vi "Get Custom Device in System Definition.vi"(8 "error in (no error)":errorcluster, 11 "system definition":path) -> (0 "error out":errorcluster, 3 "Ballard ARINC 429 custom device":u64)   [LabVIEW 2020, in "Mutation.lvclass"]
uses:
  Mutation.lvclass
  NationalInstruments.VeriStand.SystemDefinitionAPI
  <vilib>/NI/VeriStand Custom Device Testing Tools/VeriStandTestUtilities/VeriStandTestUtilities.lvlib
  Scripting/Ballard/Ballard ARINC 429 Scripting.lvlib
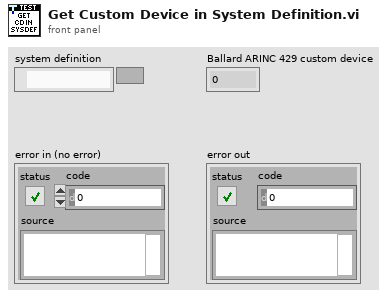
[diagram p1: front panel]
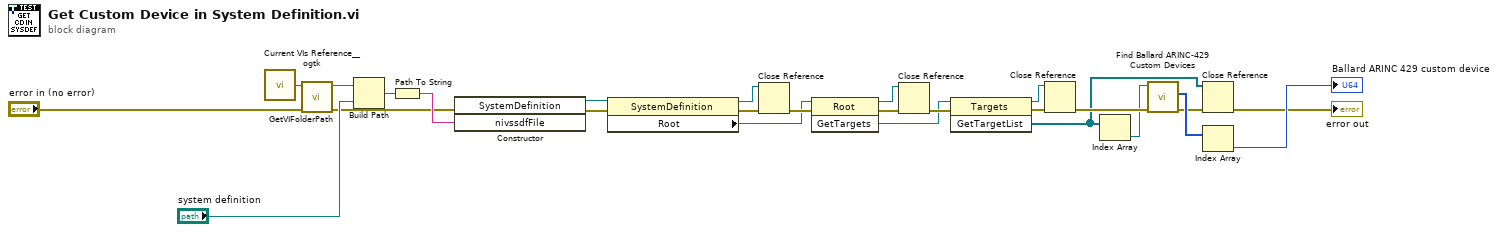
[diagram p0: block diagram]
diagram:
  n1 = call <userlib>:"Current VIs Reference__ogtk.vi"() -> ("Current VI's reference"=w1:refnum<vi>)  [unwired: 5 in]
  n2 = call <vilib>:"GetVIFolderPath.vi"("error in (no error)"="error in (no error)", "VI Reference in"=w1) -> ("error out"=w4:errorcluster, "VI Folder Path out"=w2:path)  [unwired: 8 in]
  n3 = Build Path(base path=w2, name or relative path="system definition") -> (appended path=w6:path)
  n4 = Path To String(path=w6) -> (string=w7:string)
  n5 = constructor class="SystemDefinition"(error in=w4, "nivssdfFile"=w7) -> (reference out=w10:refnum<k24>, error out=w8:errorcluster)  [unwired: 2 in, 2 out]
  n6 = property class="SystemDefinition"(reference=w10, error in=w8) -> (reference out=w22:refnum<k24>, error out=w9:errorcluster, "Root"=w11:refnum<k24>)
  n7 = Close Reference(reference=w22, error in (no error)=w9) -> (error out=w21:errorcluster)
  n8 = invoke class="Root" method="GetTargets"(reference=w11, error in=w21) -> (reference out=w20:refnum<k24>, error out=w12:errorcluster, "GetTargets"=w13:refnum<k24>)  [unwired: 1 in]
  n9 = Close Reference(reference=w20, error in (no error)=w12) -> (error out=w19:errorcluster)
  n10 = invoke class="Targets" method="GetTargetList"(reference=w13, error in=w19) -> (reference out=w18:refnum<k24>, "GetTargetList"=w16:refnum<k24>[])  [unwired: 1 in, 1 out]
  n11 = Close Reference(reference=w18, error in (no error)=w19) -> (error out=w17:errorcluster)
  n12 = Index Array(array=w16) -> (element=w14:refnum<k24>)  [unwired: 1 in]
  n13 = call "Find Ballard ARINC-429 Custom Devices.vi"("error in"=w17, "target in"=w14) -> ("error out"=w15:errorcluster, "Ballard ARINC 429 custom devices"=w23:u64[])  [unwired: 7 in, 1 out]
  n14 = Close Reference(reference=w16, error in (no error)=w15) -> (error out=→"error out":errorcluster)
  n15 = Index Array(array=w23) -> (element=→"Ballard ARINC 429 custom device":u64)  [unwired: 1 in]
